vi "sub_getNextTopLevelGuess.vi"(10 "Q2":refnum<queue>, 11 "Q1":refnum<queue>) -> (3 "q1 empty ?":bool)   [LabVIEW 2018]
uses:
  guess.ctl
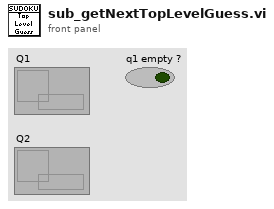
[diagram p1: front panel]
types:
  T1 = typedef "guess.ctl" = cluster{"cell position":cluster{"row":i32, "col":i32}, "guess":string}
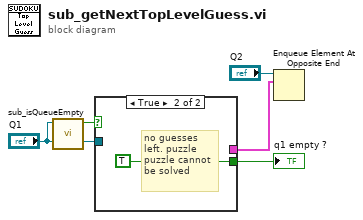
[diagram p0: block diagram]
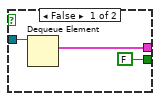
[diagram p2: hidden frame]
diagram:
  n1 = call "sub_isQueueEmpty"("Q1"="Q1") -> ("empty ?"=w1:bool)  [unwired: 10 in]
  n2 = case shown="True" w1 {
    tunnel: [FALSE TRUE] -> w2
    tunnel: "Q1" -> [w8 _]
    tunnel: [w7 _] -> w5
    frame False {
      n3 = Dequeue Element(queue=w8) -> (element=w7:T1)  [unwired: 2 in, 3 out]
    }
    frame True {
      # "no guesses\nleft. puzzle \npuzzle cannot\nbe solved"
    }
  }
  "q1 empty ?" <- w2
  n4 = Enqueue Element At Opposite End(queue="Q2", element=w5) -> ()  [unwired: 2 in, 3 out]
